vi "Initialize Software.vi"(8 "error in":errorcluster, 11 "Launcher in":refnum<class "Launcher.lvclass">) -> (0 "error out":errorcluster, 3 "Launcher out":refnum<class "Launcher.lvclass">)   [LabVIEW 2019, in "Launcher.lvlib" / "Launcher.lvclass"]
uses:
  Library/Launcher.lvclass
  Library/Launcher.lvclass/Launcher.ctl
  builds/Base Software/Base Software.lvlibp/Base Software Messages/Respond to Menu Event Msg/Respond to Menu Event Msg.lvclass
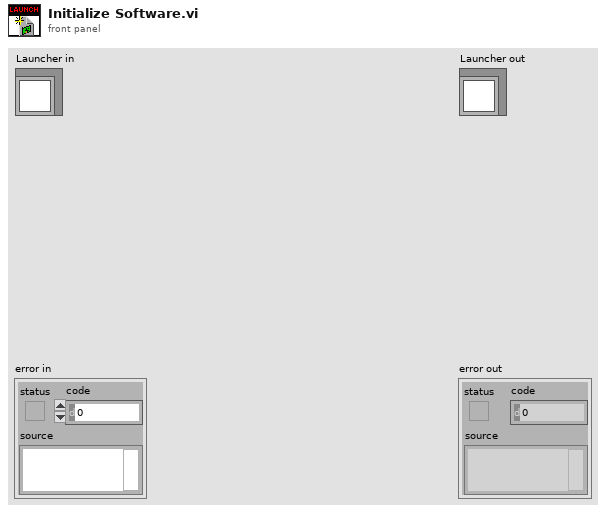
[diagram p1: front panel]
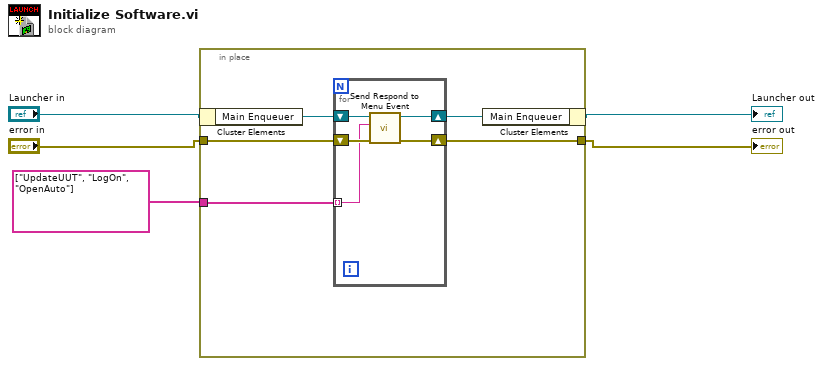
[diagram p0: block diagram]
diagram:
  n1 = in-place {
    in-place-border: [w8] -> w2
    in-place-border: "error in" -> [w7]
    in-place-border: string[] ["UpdateUUT", "LogOn", "OpenAuto"] -> [w6]
    n2 = in-place-cluster #1("Launcher in") -> ("Main Enqueuer"=w10:refnum<class "Message Enqueuer.lvclass">)
    n3 = for {
      shift-right: [w14] -> w9
      shift-left: w10 -> [w15]
      shift-right: [w13] -> w8
      shift-left: w7 -> [w12]
      tunnel: w6 -> [w11] mode=indexing
      n4 = call "Send Respond to Menu Event.vi"("error in (no error)"=w12, "Selection"=w11, "Message Enqueuer"=w15) -> ("error out"=w13:errorcluster, "Message Enqueuer out"=w14:refnum<class "Message Enqueuer.lvclass">)  [unwired: 7 in]
    }
    n5 = in-place-cluster #1("Main Enqueuer"=w9) -> (→"Launcher out":refnum<class "Launcher.lvclass">)
  }
  "error out" <- w2
